vi "SMR_LabVIEW_V6.5.vi"() -> ()   [LabVIEW 2025]
uses:
  <vilib>/DAQmx/read.llb/DAQmx Read (Analog 1D DBL NChan 1Samp).vi
  <vilib>/DAQmx/create/channels.llb/DAQmx Create Channel (AI-Temperature-Thermocouple).vi
  <vilib>/DAQmx/create/channels.llb/DAQmx Create Channel (AI-Voltage-Basic).vi
  <vilib>/DAQmx/miscellaneous.llb/DAQmx Fill In Error Info.vi
panel:
  out "Current Run Folder":path
  in  "Log Root Folder":path=path "C:/Users/LocalUser/Documents/GitHub/thermal-loop/resources/v0.1.1/data/001"
  out "Heat Exchanger Pressure History":dbl(graph)
  out "Main Loop Pressure History":T1(graph)
  out "Heat Exchanger Temperature History":cluster{"Waveform":dbl, "Waveform":dbl}(graph)
  out "Main Loop Temeperature History":T2(graph)
  out "Overall Avg Pressure (psi)":dbl
  out "Heat Exchanger Pressure P6 (psi)":dbl
  out "Main Loop Avg Pressure (psi)":dbl
  out "Heat Exchanger Avg Temp (deg C)":dbl
  out "Main Loop Avg Temp (deg C)":dbl
  out "Raw NI9201 \nVoltage Display":T3
  out "Temperature Display":T4
  out "Pressure Display":T5
  in  "Flow Offset Correction (GPM)":dbl=-0.3
  out "Flow History":dbl(graph)
  out "Overall Pressure History":T6(graph)
  out "Overall Temperature History":T7(graph)
  out "Max Loop Pressure (psi)":dbl
  out "Overall Avg Temp (deg C)":dbl
  out "Max Loop Temp (deg C)":dbl
  out "Heat Exchanger Flow (GPM)":dbl
  in  "Loop Period (ms)":dbl=1000.0
  in  "Stop":bool
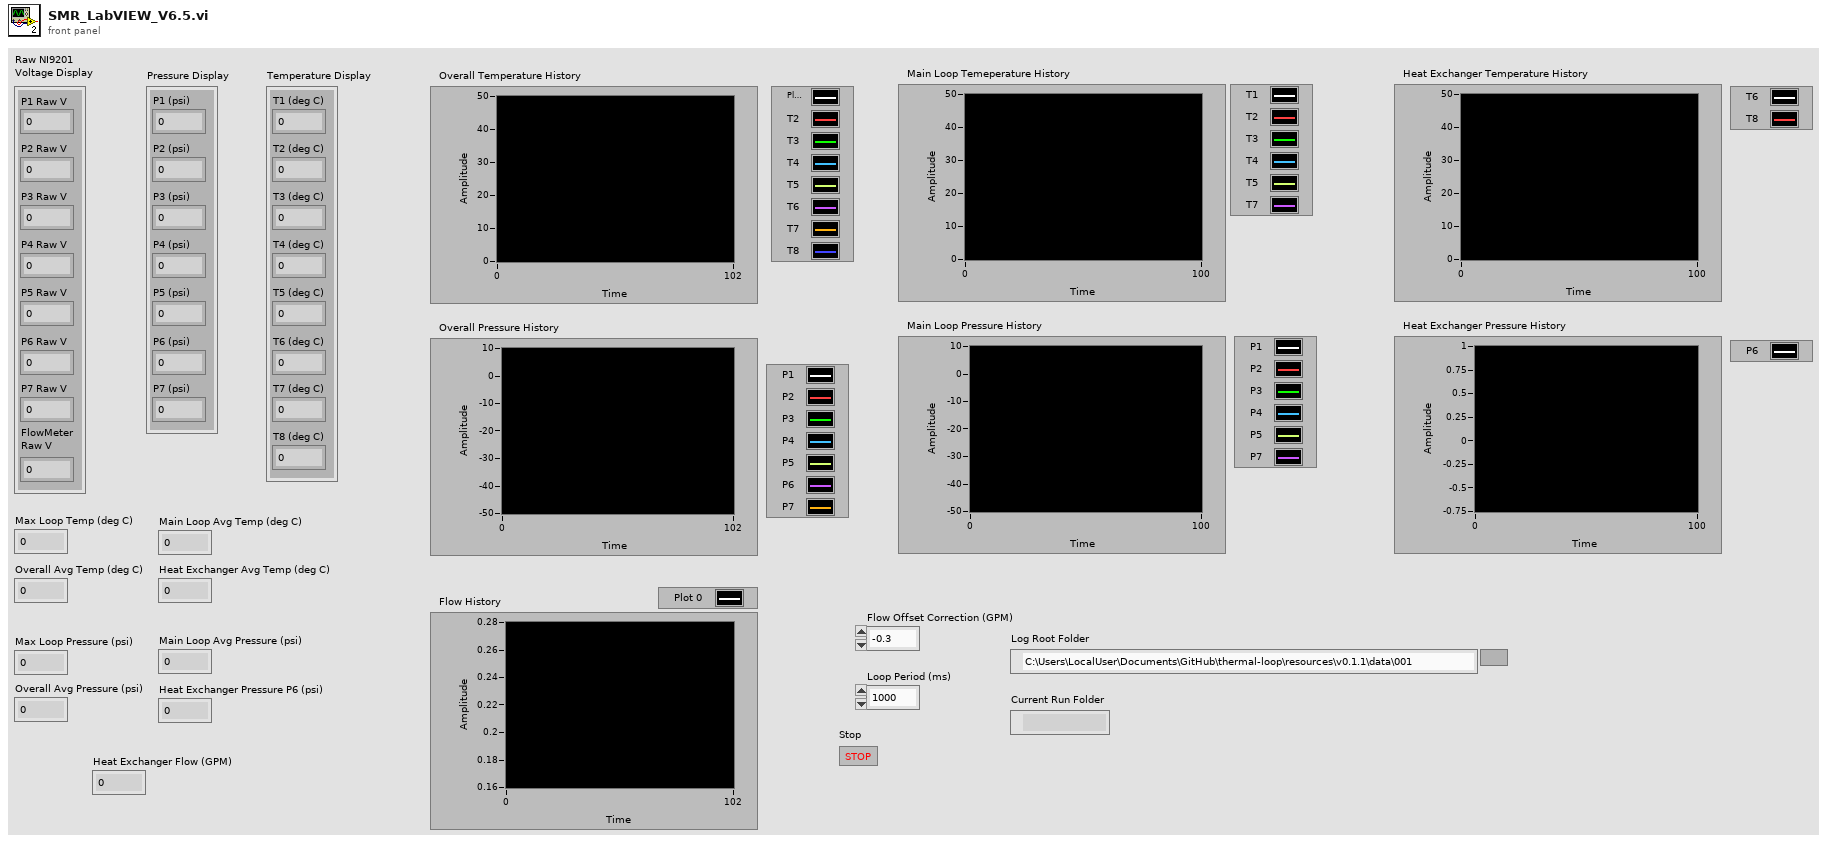
[diagram p1: front panel]
types:
  T1 = cluster{"P1":dbl, "P2":dbl, "P3":dbl, "P4":dbl, "P5":dbl, "P7":dbl}
  T2 = cluster{"Waveform":dbl, "Waveform":dbl, "Waveform":dbl, "Waveform":dbl, "Waveform":dbl, "Waveform":dbl}
  T3 = cluster{"P1 Raw V":dbl, "P2 Raw V":dbl, "P3 Raw V":dbl, "P4 Raw V":dbl, "P5 Raw V":dbl, "P6 Raw V":dbl, "P7 Raw V":dbl, "FlowMeter\nRaw V":dbl}
  T4 = cluster{"T1 (deg C)":dbl, "T2 (deg C)":dbl, "T3 (deg C)":dbl, "T4 (deg C)":dbl, "T5 (deg C)":dbl, "T6 (deg C)":dbl, "T7 (deg C)":dbl, "T8 (deg C)":dbl}
  T5 = cluster{"P1 (psi)":dbl, "P2 (psi)":dbl, "P3 (psi)":dbl, "P4 (psi)":dbl, "P5 (psi)":dbl, "P6 (psi)":dbl, "P7 (psi)":dbl}
  T6 = cluster{"P1":dbl, "P2":dbl, "P3":dbl, "P4":dbl, "P5":dbl, "P6":dbl, "P7":dbl}
  T7 = cluster{"Waveform":dbl, "Waveform":dbl, "Waveform":dbl, "Waveform":dbl, "Waveform":dbl, "Waveform":dbl, "Waveform":dbl, "Waveform":dbl}
  T8 = enum16{"open", "replace", "create", "open or create", "replace or create", "replace or create with confirmation"}
  T9 = cluster{"P1":dbl, "P2":dbl, "P3":dbl, "P4":dbl, "P5":dbl, "P6":dbl, "P7":dbl, "Flow":dbl}
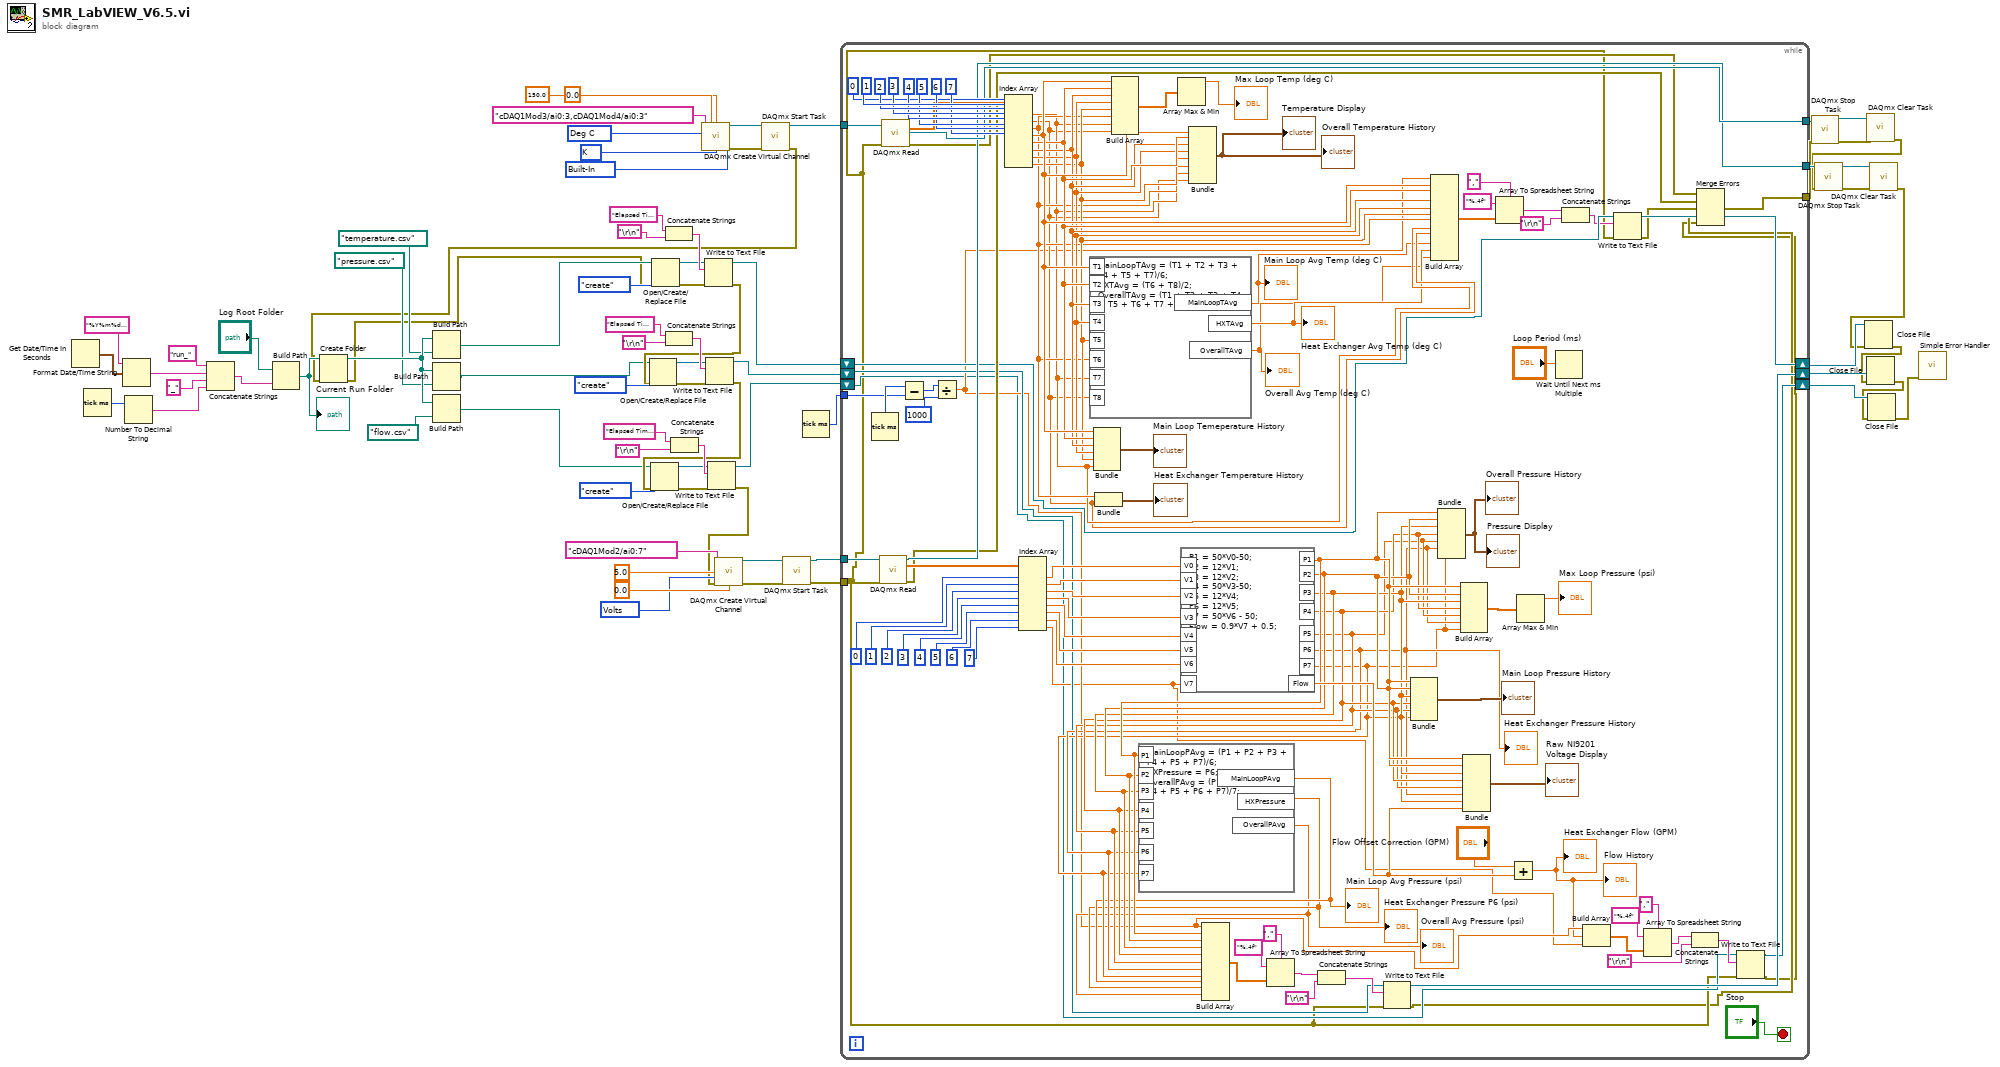
[diagram p0: block diagram]
diagram:
  w64 = 10200 items=["Built-In"=10200, "Constant Value"=10116, "Channel"=10113] ("cjc source")
  w65 = 10073 items=["J"=10072, "K"=10073, "N"=10077, "R"=10082, "S"=10085, "T"=10086, "B"=10047, "E"=10055] ("thermocouple type")
  w66 = 10143 items=["Deg C"=10143, "Deg F"=10144, "Kelvins"=10325, "Deg R"=10145, "From Custom Scale"=10065] ("units")
  w73 = 10348 items=["Volts"=10348, "From Custom Scale"=10065] ("units")
  n1 = Get Date/Time In Seconds() -> (seconds since 1Jan1904=w19:timestamp)
  n2 = Tick Count (ms)() -> (millisecond timer value=w17:u32)
  n3 = Format Date/Time String(time format string (%c)="%Y%m%d_%H%M%S", seconds (now)=w19) -> (date/time string=w14:string)  [unwired: 1 in]
  n4 = Number To Decimal String(number=w17) -> (decimal integer string=w15:string)  [unwired: 1 in]
  n5 = Concatenate Strings("run_" ("string"), w14, "_" ("string"), w15) -> (w11:string)
  n6 = Build Path(base path="Log Root Folder", name or relative path=w11) -> (appended path=w10:path)
  "Current Run Folder" <- w10
  n7 = Concatenate Strings("Elapsed Time (s),T1 (deg C),T2 (deg C),T3 (deg C),T4 (deg C),T5 (deg C),T6 (deg C),T7 (deg C),T8 (deg C),Main Loop Avg Temp (deg C),HX Avg Temp (deg C),Overall Avg Temp (deg C)", "\r\n") -> (w46:string)
  n8 = Concatenate Strings("Elapsed Time (s),P1 (psi),P2 (psi),P3 (psi),P4 (psi),P5 (psi),P6 (psi),P7 (psi),Main Loop Avg Pressure (psi),HX Pressure (psi),Overall Avg Pressure (psi)", "\r\n") -> (w44:string)
  n9 = Concatenate Strings("Elapsed Time (s),Heat Exchanger Flow (GPM),Flow Raw Voltage (V)", "\r\n") -> (w40:string)
  n10 = call-poly <vilib>:"DAQmx Create Virtual Channel.vi"("maximum value"=150.0, "minimum value"=0.0, "physical channels"=tag "cDAQ1Mod3/ai0:3,cDAQ1Mod4/ai0:3", "cjc source"=w64, "units"=w66, "thermocouple type"=w65) -> ("task out"=w63:refnum<k21>, "error out"=w62:errorcluster)  [unwired: 8 in]
  n11 = call <vilib>:"DAQmx Start Task.vi"("task/channels in"=w63, "error in"=w62) -> ("task out"=w61:refnum<k21>, "error out"=w2:errorcluster)  [unwired: 12 in]
  n12 = Create Folder(path (use dialog)=w10, error in=w2) -> (created path=w9:path, error out=w1:errorcluster)  [unwired: 1 in, 1 out]
  n13 = Build Path(base path=w9, name or relative path=path "temperature.csv") -> (appended path=w8:path)
  n14 = Build Path(base path=w9, name or relative path=path "pressure.csv") -> (appended path=w7:path)
  n15 = Build Path(base path=w9, name or relative path=path "flow.csv") -> (appended path=w6:path)
  n16 = Open/Create/Replace File(file path (use dialog)=w8, error in=w1, operation (0:open)=T8."create") -> (refnum out=w45:refnum<file>, error out=w29:errorcluster)  [unwired: 3 in, 1 out]
  n17 = Write to Text File(file (use dialog)=w45, text=w46, error in=w29) -> (refnum out=w36:refnum<file>, error out=w28:errorcluster)  [unwired: 1 in, 1 out]
  n18 = Open/Create/Replace File(file path (use dialog)=w7, error in=w28, operation (0:open)=T8."create") -> (refnum out=w43:refnum<file>, error out=w27:errorcluster)  [unwired: 3 in, 1 out]
  n19 = Write to Text File(file (use dialog)=w43, text=w44, error in=w27) -> (refnum out=w35:refnum<file>, error out=w26:errorcluster)  [unwired: 1 in, 1 out]
  n20 = Open/Create/Replace File(file path (use dialog)=w6, error in=w26, operation (0:open)=T8."create") -> (refnum out=w39:refnum<file>, error out=w25:errorcluster)  [unwired: 3 in, 1 out]
  n21 = Write to Text File(file (use dialog)=w39, text=w40, error in=w25) -> (refnum out=w34:refnum<file>, error out=w24:errorcluster)  [unwired: 1 in, 1 out]
  n22 = call-poly <vilib>:"DAQmx Create Virtual Channel.vi"("maximum value"=5.0, "minimum value"=0.0, "physical channels"=tag "cDAQ1Mod2/ai0:7", "units"=w73, "error in"=w24) -> ("task out"=w72:refnum<k21>, "error out"=w71:errorcluster)  [unwired: 9 in]
  n23 = call <vilib>:"DAQmx Start Task.vi"("task/channels in"=w72, "error in"=w71) -> ("task out"=w70:refnum<k21>, "error out"=w59:errorcluster)  [unwired: 12 in]
  n24 = Tick Count (ms)() -> (millisecond timer value=w33:u32)
  n25 = while {
    tunnel: w70 -> [w174]
    tunnel: w61 -> [w147]
    tunnel: [w137] -> w60
    tunnel: w59 -> [w80]
    tunnel: [w136] -> w58
    tunnel: [w133] -> w57
    shift-right: [w111] -> w32
    shift-left: w36 -> [w112]
    shift-right: [w92] -> w31
    shift-left: w35 -> [w93]
    shift-right: [w81] -> w30
    shift-left: w34 -> [w82]
    tunnel: w33 -> [w131]
    stop <- "Stop" stop-if-true
    n26 = Tick Count (ms)() -> (millisecond timer value=w132:u32)
    n27 = call-poly <vilib>:"DAQmx Read.vi"("task/channels in"=w174, "error in"=w80) -> ("task out"=w136:refnum<k21>, "data"=w165:dbl[], "error out"=w134:errorcluster)  [unwired: 11 in]
    n28 = call-poly <vilib>:"DAQmx Read.vi"("task/channels in"=w147, "error in"=w80) -> ("task out"=w137:refnum<k21>, "data"=w138:dbl[], "error out"=w135:errorcluster)  [unwired: 11 in]
    n29 = Subtract(x=w132, y=w131) -> (x-y=w130:u32)
    n30 = Divide(x=w130, y=u32 1000) -> (x/y=w91:dbl)
    n31 = Index Array(array=w138, index #1=0 ("index"), index #2=1 ("index"), index #3=2 ("index"), index #4=3 ("index"), index #5=4 ("index"), index #6=5 ("index"), index #7=6 ("index"), index #8=7 ("index")) -> (element #1=w122:dbl, element #2=w121:dbl, element #3=w123:dbl, element #4=w128:dbl, element #5=w127:dbl, element #6=w126:dbl, element #7=w125:dbl, element #8=w124:dbl)
    n32 = Index Array(array=w165, index #1=0 ("index"), index #2=1 ("index"), index #3=2 ("index"), index #4=3 ("index"), index #5=4 ("index"), index #6=5 ("index"), index #7=6 ("index"), index #8=7 ("index")) -> (element #1=w164:dbl, element #2=w163:dbl, element #3=w162:dbl, element #4=w161:dbl, element #5=w160:dbl, element #6=w159:dbl, element #7=w158:dbl, element #8=w89:dbl)
    n33 = formula code="MainLoopTAvg = (T1 + T2 + T3 + T4 + T5 + T7)/6;\nHXTAvg = (T6 + T8)/2;\nOverallTAvg = (T1 + T2 + T3 + T4 + T5 + T6 + T7 + T8)/8;"("T1"=w128, "T2"=w127, "T3"=w126, "T4"=w125, "T5"=w124, "T6"=w123, "T7"=w122, "T8"=w121) -> ("MainLoopTAvg"=w120:dbl, "HXTAvg"=w119:dbl, "OverallTAvg"=w118:dbl)
    "Overall Avg Temp (deg C)" <- w118
    "Main Loop Avg Temp (deg C)" <- w120
    "Heat Exchanger Avg Temp (deg C)" <- w119
    n34 = Bundle("Waveform"=w128, "Waveform"=w127, "Waveform"=w126, "Waveform"=w125, "Waveform"=w124, "Waveform"=w122) -> (→"Main Loop Temeperature History":T2)  [unwired: 1 in]
    n35 = Bundle("Waveform"=w123, "Waveform"=w121) -> (→"Heat Exchanger Temperature History":cluster{"Waveform":dbl, "Waveform":dbl})  [unwired: 1 in]
    n36 = Build Array(w128, w127, w126, w125, w124, w123, w122, w121) -> (w175:dbl[])
    n37 = Array Max & Min(array=w175) -> (max value=→"Max Loop Temp (deg C)":dbl)  [unwired: 3 out]
    n38 = formula code="P1 = 50*V0-50;\nP2 = 12*V1;\nP3 = 12*V2;\nP4 = 50*V3-50;\nP5 = 12*V4;\nP6 = 12*V5; \nP7 = 50*V6 - 50;\nFlow = 0.9*V7 + 0.5;"("V0"=w164, "V1"=w163, "V2"=w162, "V3"=w161, "V4"=w160, "V5"=w159, "V6"=w158, "V7"=w89) -> ("P1"=w110:dbl, "P2"=w109:dbl, "P3"=w108:dbl, "P4"=w107:dbl, "P5"=w106:dbl, "P6"=w105:dbl, "P7"=w104:dbl, "Flow"=w152:dbl)
    "Heat Exchanger Pressure History" <- w105
    n39 = formula code="MainLoopPAvg = (P1 + P2 + P3 + P4 + P5 + P7)/6;\nHXPressure = P6;\nOverallPAvg = (P1 + P2 + P3 + P4 + P5 + P6 + P7)/7;"("P1"=w110, "P2"=w109, "P3"=w108, "P4"=w107, "P5"=w106, "P6"=w105, "P7"=w104) -> ("MainLoopPAvg"=w103:dbl, "HXPressure"=w102:dbl, "OverallPAvg"=w101:dbl)
    "Overall Avg Pressure (psi)" <- w101
    "Heat Exchanger Pressure P6 (psi)" <- w102
    "Main Loop Avg Pressure (psi)" <- w103
    n40 = Bundle("Waveform"=w128, "Waveform"=w127, "Waveform"=w126, "Waveform"=w125, "Waveform"=w124, "Waveform"=w123, "Waveform"=w122, "Waveform"=w121) -> (→"Overall Temperature History" →"Temperature Display":T7)  [unwired: 1 in]
    n41 = Build Array(w91, w110, w109, w108, w107, w106, w105, w104, w103, w102, w101) -> (w100:dbl[])
    n42 = Array To Spreadsheet String(delimiter (Tab)=",", array=w100, 3:"%.4f" ("format string")) -> (spreadsheet string=w96:string)
    n43 = Concatenate Strings(w96, "\r\n") -> (w94:string)
    n44 = Write to Text File(file (use dialog)=w93, text=w94, error in=w80) -> (refnum out=w92:refnum<file>, error out=w78:errorcluster)  [unwired: 1 in, 1 out]
    n45 = Bundle("P1"=w110, "P2"=w109, "P3"=w108, "P4"=w107, "P5"=w106, "P7"=w104) -> (→"Main Loop Pressure History":T1)  [unwired: 1 in]
    n46 = Build Array(w91, w128, w127, w126, w125, w124, w123, w122, w121, w120, w119, w118) -> (w117:dbl[])
    n47 = Bundle("P1"=w110, "P2"=w109, "P3"=w108, "P4"=w107, "P5"=w106, "P6"=w105, "P7"=w104) -> (→"Overall Pressure History" →"Pressure Display":T6)  [unwired: 1 in]
    n48 = Build Array(w110, w109, w108, w107, w106, w105, w104) -> (w155:dbl[])
    n49 = Bundle("P1"=w110, "P2"=w109, "P3"=w108, "P4"=w107, "P5"=w106, "P6"=w105, "P7"=w104, "Flow"=w152) -> (→"Raw NI9201 \nVoltage Display":T9)  [unwired: 1 in]
    n50 = Array To Spreadsheet String(delimiter (Tab)=",", array=w117, 3:"%.4f" ("format string")) -> (spreadsheet string=w114:string)
    n51 = Add(x="Flow Offset Correction (GPM)", y=w152) -> (x+y=w90:dbl)
    "Heat Exchanger Flow (GPM)" <- w90
    "Flow History" <- w90
    n52 = Array Max & Min(array=w155) -> (max value=→"Max Loop Pressure (psi)":dbl)  [unwired: 3 out]
    n53 = Wait Until Next ms Multiple(millisecond multiple="Loop Period (ms)") -> ()  [unwired: 1 out]
    n54 = Concatenate Strings(w114, "\r\n") -> (w97:string)
    n55 = Build Array(w91, w90, w89) -> (w88:dbl[])
    n56 = Write to Text File(file (use dialog)=w112, text=w97, error in=w80) -> (refnum out=w111:refnum<file>, error out=w79:errorcluster)  [unwired: 1 in, 1 out]
    n57 = Array To Spreadsheet String(delimiter (Tab)=",", array=w88, 3:"%.4f" ("format string")) -> (spreadsheet string=w84:string)
    n58 = Concatenate Strings(w84, "\r\n") -> (w83:string)
    n59 = Write to Text File(file (use dialog)=w82, text=w83, error in=w80) -> (refnum out=w81:refnum<file>, error out=w77:errorcluster)  [unwired: 1 in, 1 out]
    n60 = Merge Errors(w135, w134, w79, w78, w77) -> (w133:errorcluster)
  }
  n61 = call <vilib>:"DAQmx Stop Task.vi"("task/channels in"=w60, "error in"=w57) -> ("task out"=w56:refnum<k21>, "error out"=w54:errorcluster)  [unwired: 12 in]
  n62 = call <vilib>:"DAQmx Clear Task.vi"("task in"=w56, "error in"=w54) -> ("error out"=w53:errorcluster)  [unwired: 13 in]
  n63 = call <vilib>:"DAQmx Stop Task.vi"("task/channels in"=w58, "error in"=w53) -> ("task out"=w55:refnum<k21>, "error out"=w52:errorcluster)  [unwired: 12 in]
  n64 = call <vilib>:"DAQmx Clear Task.vi"("task in"=w55, "error in"=w52) -> ("error out"=w23:errorcluster)  [unwired: 13 in]
  n65 = Close File(refnum=w32, error in=w23) -> (error out=w22:errorcluster)  [unwired: 1 out]
  n66 = Close File(refnum=w31, error in=w22) -> (error out=w21:errorcluster)  [unwired: 1 out]
  n67 = Close File(refnum=w30, error in=w21) -> (error out=w20:errorcluster)  [unwired: 1 out]
  n68 = call <vilib>:"Simple Error Handler.vi"("error in (no error)"=w20) -> ()  [unwired: 4 in, 5 out]
